vi "GetGrabberPositions.vi"(0 "reference":refnum<class "NoteNode.lvclass">, 5 "error in (no error)":errorcluster) -> (14 "reference out":refnum<class "NoteNode.lvclass">, 15 "GrabberPositions":T2[](array[typedef]) {"y" format="%.2f"; "x" format="%.2f"}, 16 "HotSpots":T1[](array[typedef]) {"HotSpot"."y" format="%.2f"; "HotSpot"."x" format="%.2f"}, 19 "error out":errorcluster)   [LabVIEW 2020, in "NoteNode.lvclass"]
doc: "public Rectangle2D getBounds(Graphics2D g2)"
uses:
  <resource>/Framework/Providers/Open_GDS/UML/NoteNode_class/NoteNode.lvclass
  C:/Program Files (x86)/National Instruments/LabVIEW 2020/resource/Framework/Providers/Open_GDS/UML/AbstractNode_class/AbstractNode.lvclass
  <resource>/Framework/Providers/Open_GDS/UML/General/Point/Point Point2D.ctl
  <resource>/Framework/Providers/Open_GDS/UML/UMLEditor/UMLEditor_HotSpotData.ctl
  <resource>/Framework/Providers/Open_GDS/UML/AbstractNode_class/AbstractNode.lvclass
  <resource>/Framework/Providers/Open_GDS/UML/UMLEditor/UMLEditor_HotSpotType.ctl
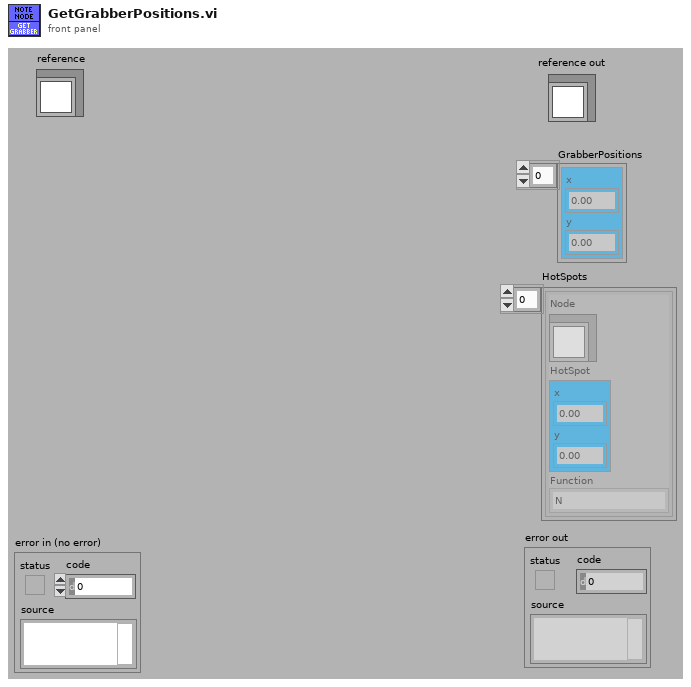
[diagram p1: front panel]
types:
  T1 = typedef "UMLEditor_HotSpotData.ctl" = cluster{"Node":refnum<class "AbstractNode.lvclass">, "HotSpot":T2, "Function":T3}
  T2 = typedef "Point Point2D.ctl" = cluster{"x":dbl, "y":dbl}
  T3 = typedef "UMLEditor_HotSpotType.ctl" = enum16{"N", "NE", "E", "SE", "S", "SW", "W", "NW", "Expand", "Collaps"}
  T4 = typedef "Rectangle Rectangle2D.ctl" = cluster{"x":dbl, "y":dbl, "width":dbl, "height":dbl}
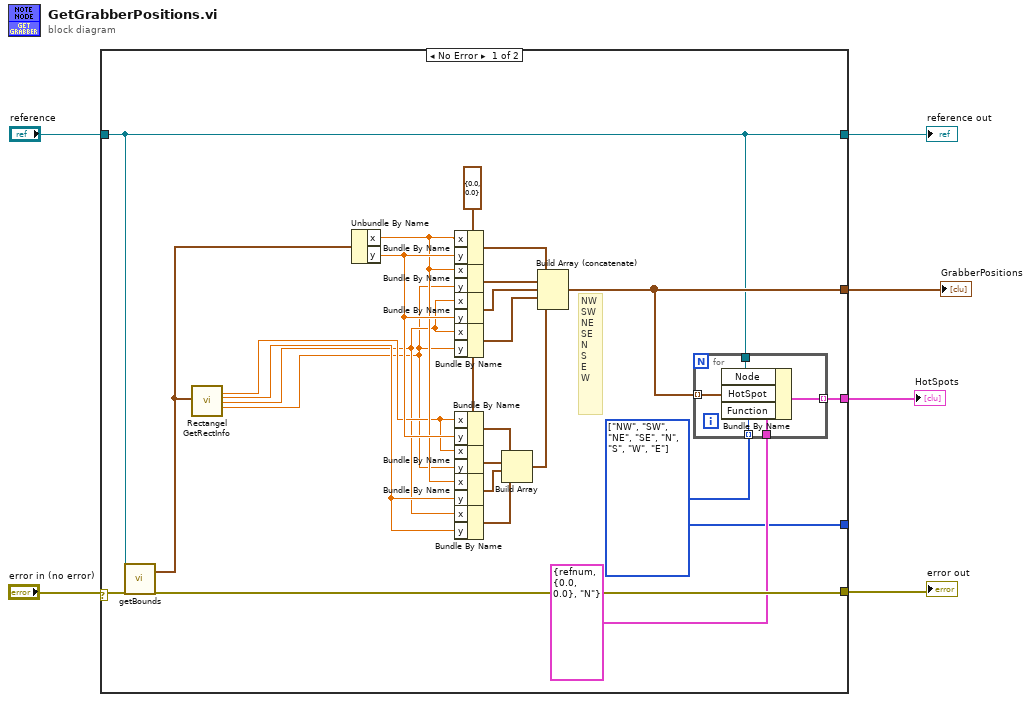
[diagram p0: block diagram]
diagram:
  n1 = case shown="No Error" "error in (no error)" {
    selector: "error in (no error)" -> [w19 w36]
    tunnel: "reference" -> [w7 w37]
    tunnel: [w18 w36] -> w5
    tunnel: [w7 w37] -> w4
    tunnel: [w8 _] -> w2
    tunnel: [w9 _] -> _
    tunnel: [w10 _] -> w1
    frame No Error {
      w9 = T3[] [enum."NW", enum."SW", enum."NE", enum."SE", enum."N", enum."S", enum."W", enum."E"] items=["N", "NE", "E", "SE", "S", "SW", "W", "NW", "Expand", "Collaps"]
      w12 = T2 {"x"=0.0, "y"=0.0} ("point2D")
      # "NW\nSW\nNE\nSE\nN\nS\nE\nW"
      n2 = call-dynamic "getBounds.vi"("reference"=w7, "error in (no error)"=w19) -> ("bounds"=w17:T4, "error out"=w18:errorcluster)  [unwired: 15 in, 1 out]
      n3 = call <resource>:"Rectangel GetRectInfo.vi"("bounds"=w17) -> ("centerX"=w16:dbl, "centerY"=w15:dbl, "maxX"=w14:dbl, "maxY"=w13:dbl)  [unwired: 1 in, 14 out]
      n4 = Unbundle By Name(w17) -> ("x"=w20:dbl, "y"=w22:dbl)
      n5 = Bundle By Name(cluster=w12, "x"=w20, "y"=w22) -> (w30:T2)
      n6 = Bundle By Name(cluster=w12, "x"=w20, "y"=w13) -> (w29:T2)
      n7 = Bundle By Name(cluster=w12, "x"=w14, "y"=w22) -> (w28:T2)
      n8 = Bundle By Name(cluster=w12, "x"=w14, "y"=w13) -> (w27:T2)
      n9 = Bundle By Name(cluster=w12, "x"=w16, "y"=w22) -> (w23:T2)
      n10 = Bundle By Name(cluster=w12, "x"=w16, "y"=w13) -> (w24:T2)
      n11 = Bundle By Name(cluster=w12, "x"=w20, "y"=w15) -> (w25:T2)
      n12 = Bundle By Name(cluster=w12, "x"=w14, "y"=w15) -> (w26:T2)
      n13 = Build Array(w23, w24, w25, w26) -> (w21:T2[])
      n14 = Build Array (concatenate)(w30, w29, w28, w27, w21) -> (w8:T2[])
      n15 = for {
        tunnel: T1 {"Node"=refnum, "HotSpot"={"x"=0.0, "y"=0.0}, "Function"=enum."N"} ("ObjectHotSpot") -> [w35]
        tunnel: [w34] -> w10 mode=indexing
        tunnel: w9 -> [w33] mode=indexing
        tunnel: w8 -> [w32] mode=indexing
        tunnel: w7 -> [w31]
        n16 = Bundle By Name(cluster=w35, "Node"=w31, "HotSpot"=w32, "Function"=w33) -> (w34:T1)
      }
    }
    frame Error {
    }
  }
  "reference out" <- w4
  "error out" <- w5
  "GrabberPositions" <- w2
  "HotSpots" <- w1
